vi "Uninit.vi"(2 "Container State":T1, 3 "Display State":T2) -> ()   [LabVIEW 2021, in "Clock.xctl"]
uses:
  Clock.xctl
  State.ctl
  <resource>/importtools/Common/Event/NISAST Event.lvclass
  <vilib>/_xctls/Container State.ctl
  <vilib>/_xctls/XControlSupport.lvlib
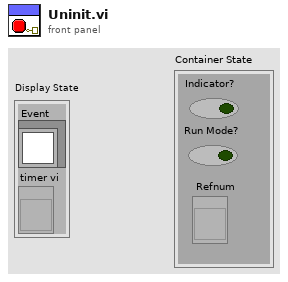
[diagram p1: front panel]
types:
  T1 = typedef "XControlSupport.lvlib/Container State.ctl" = cluster{"Indicator?":bool, "Run Mode?":bool, " Refnum":refnum<vi>}
  T2 = typedef "Clock.xctl/State.ctl" = cluster{"Event":refnum<class "NISAST Event.lvclass">, "timer vi":refnum<vi>}
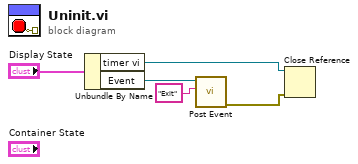
[diagram p0: block diagram]
diagram:
  n1 = Unbundle By Name("Display State") -> ("timer vi"=w2:refnum<vi>, "Event"=w4:refnum<class "NISAST Event.lvclass">)
  n2 = call-dynamic "Post Event.vi"("Event Name"="Exit", "Event in"=w4) -> ("error out"=w1:errorcluster)  [unwired: 8 in, 1 out]
  n3 = Close Reference(reference=w2, error in (no error)=w1) -> ()  [unwired: 1 out]
